vi "PH_Beckhoff_PP_PU.set i Attr and start DIM Services for PSU.vi"(0 "PU Type":T4=enum."PA 19mm", 1 "PSU Info":T1, 2 "Values":T5, 3 "error in":errorcluster) -> (6 "PSU":T3(array[cluster]) {"Status"."Status" items=["no info", "off/false/out", "on/true/in", "Failure", "Alarm", "Status 1", "Status 2", "Status 3"]}, 7 "error out":errorcluster)   [LabVIEW 2014, in "PH_Beckhoff_PP_PU.lvlib"]
uses:
  PH_Beckhoff_PP_PU.lvlib
  PH_Beckhoff/PH_Beckhoff.Values.ctl
  PH_Beckhoff/PH_Beckhoff.Sonderklemmen Inputs.ctl
  PH_Beckhoff/PH_Beckhoff.Analog Inputs.ctl
  PH_Beckhoff/PH_Beckhoff.Scaling Type.ctl
  PH_Beckhoff/PH_Beckhoff.Analog Outputs.ctl
  PH_Beckhoff/PH_Beckhoff.Digital Inputs.ctl
  PH_Beckhoff/PH_Beckhoff.Digital Outputs.ctl
  PH_Beckhoff_PP_PU.PU Rack Type.ctl
  PH_Basics/PH_StatusHandler/PH_StatusHandler.Status.ctl
  PH_Basics/PH_PP_Common/PH_PP_Common.PSU Tags.ctl
  CSlibraries-extern/DimLVEvent/LVDimInterface/LVDimInterface.lvlib
  PH_Basics/PH_StatusHandler/PH_StatusHandler.lvlib
  PH_Basics/PH_PP_Common/PH_PP_Common.lvlib
  PH_Beckhoff/PH_Beckhoff.lvlib
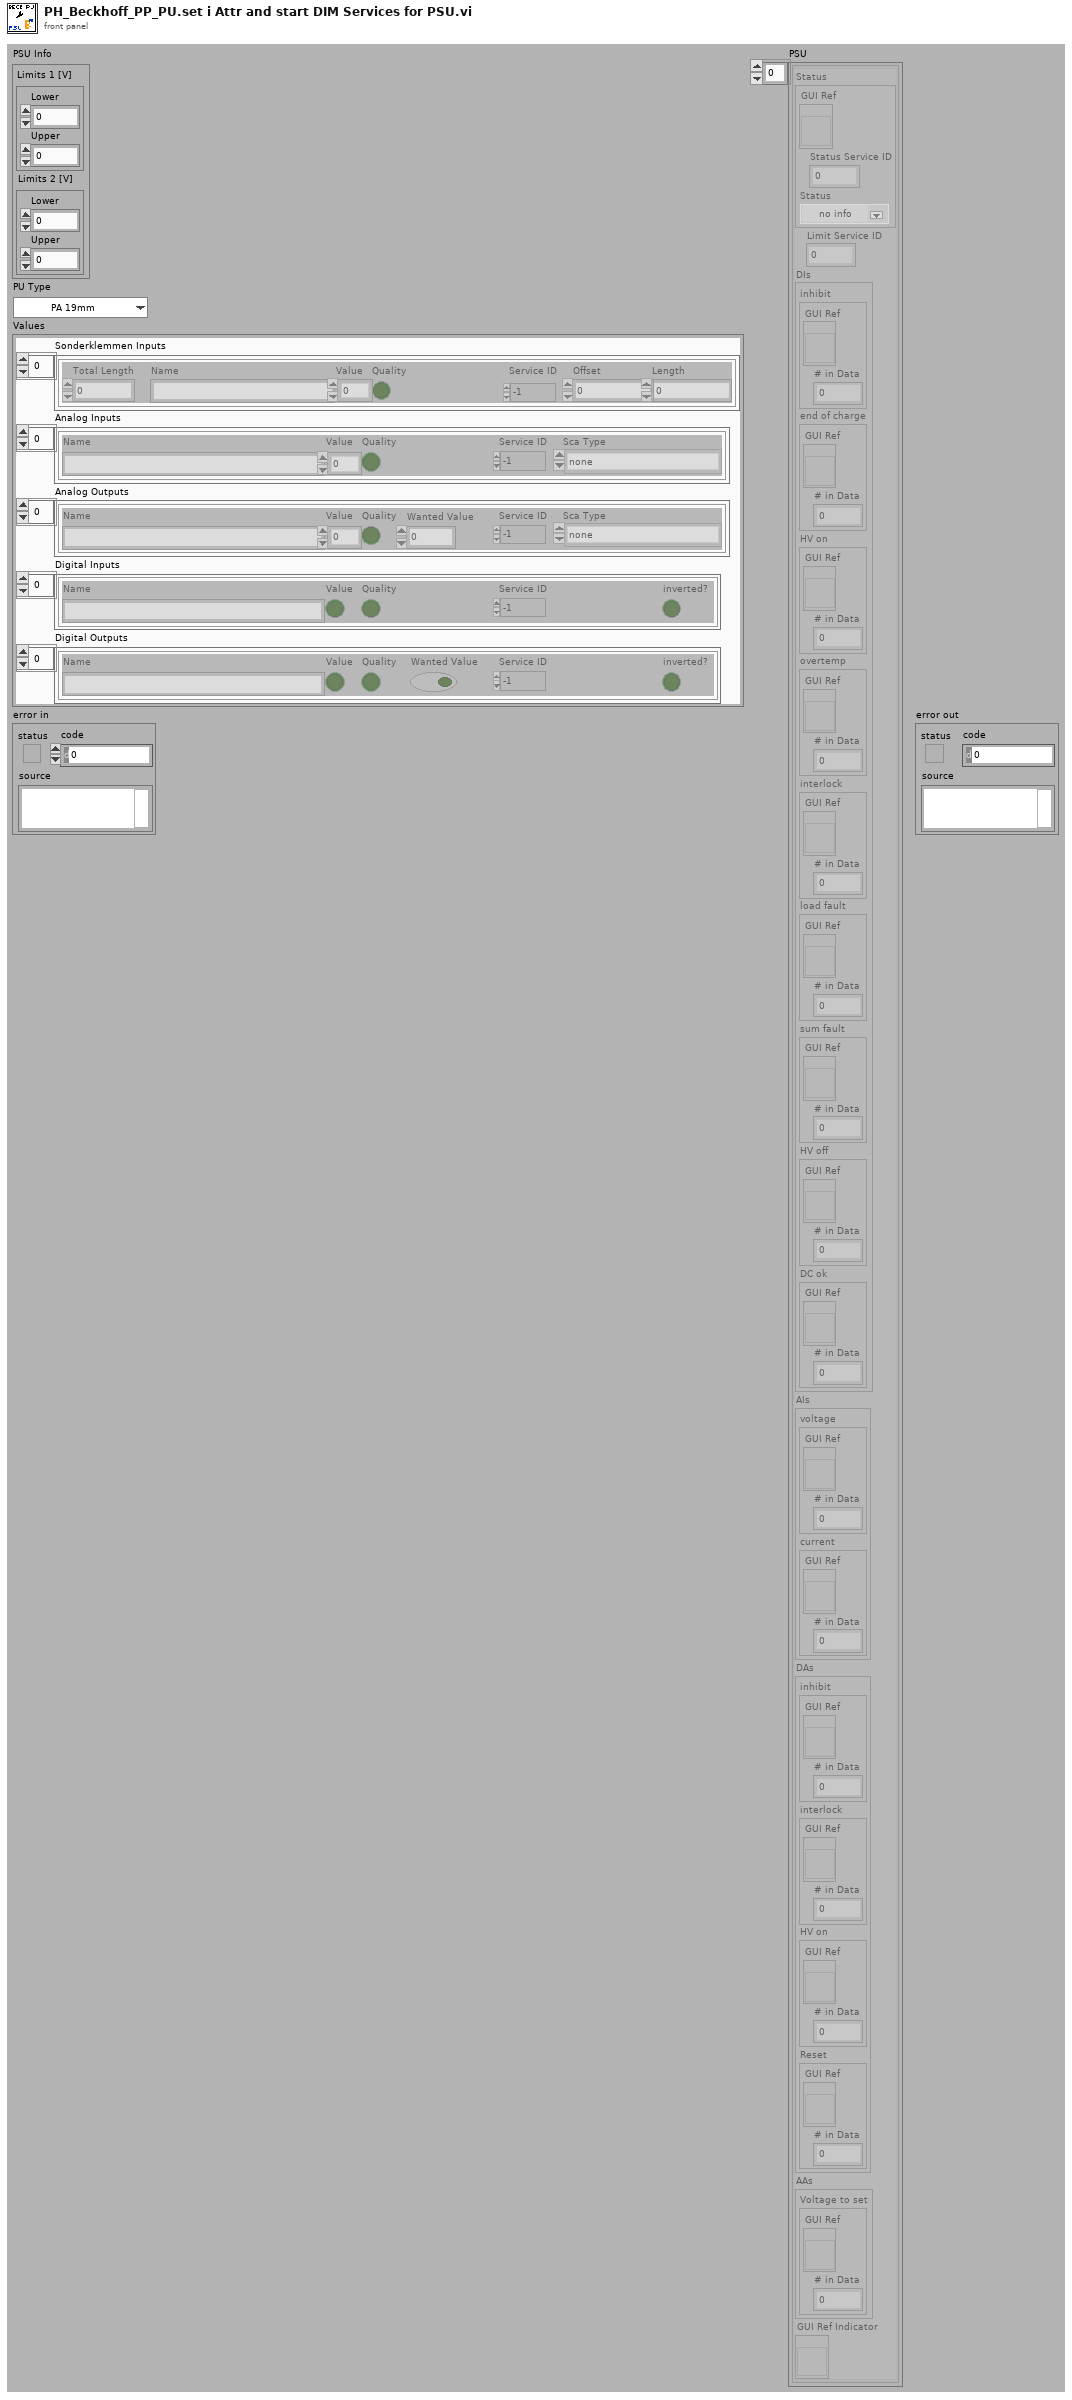
[diagram p1: front panel]
types:
  T1 = cluster{"Limits 1 [V]":cluster{"Lower":dbl, "Upper":dbl}, "Limits 2 [V]":cluster{"Lower":dbl, "Upper":dbl}}
  T2 = typedef "PH_StatusHandler.lvlib/PH_StatusHandler.Status.ctl" = i16
  T3 = cluster{"Status":cluster{"GUI Ref":refnum<vi>, "Status Service ID":i32, "Status":T2}, "Limit Service ID":i32, "DIs":cluster{"inhibit":cluster{"GUI Ref":refnum<vi>, "# in Data":i32}, "end of charge":cluster{"GUI Ref":refnum<vi>, "# in Data":i32}, "HV on":cluster{"GUI Ref":refnum<vi>, "# in Data":i32}, "overtemp":cluster{"GUI Ref":refnum<vi>, "# in Data":i32}, "interlock":cluster{"GUI Ref":refnum<vi>, "# in Data":i32}, "load fault":cluster{"GUI Ref":refnum<vi>, "# in Data":i32}, "sum fault":cluster{"GUI Ref":refnum<vi>, "# in Data":i32}, "HV off":cluster{"GUI Ref":refnum<vi>, "# in Data":i32}, "DC ok":cluster{"GUI Ref":refnum<vi>, "# in Data":i32}}, "AIs":cluster{"voltage":cluster{"GUI Ref":refnum<vi>, "# in Data":i32}, "current":cluster{"GUI Ref":refnum<vi>, "# in Data":i32}}, "DAs":cluster{"inhibit":cluster{"GUI Ref":refnum<vi>, "# in Data":i32}, "interlock":cluster{"GUI Ref":refnum<vi>, "# in Data":i32}, "HV on":cluster{"GUI Ref":refnum<vi>, "# in Data":i32}, "Reset":cluster{"GUI Ref":refnum<vi>, "# in Data":i32}}, "AAs":cluster{"Voltage to set":cluster{"GUI Ref":refnum<vi>, "# in Data":i32}}, "GUI Ref Indicator":refnum<vi>}[]
  T4 = typedef "PH_Beckhoff_PP_PU.lvlib/PH_Beckhoff_PP_PU.PU Rack Type.ctl" = enum16{"no Info", "PA 19mm", "PA 45mm", "MA PU 1 and 2", "MA PU 3 and 4", "MA PU 5 and 6", "MA FR and PILC"}
  T5 = typedef "PH_Beckhoff.lvlib/PH_Beckhoff.Values.ctl" = cluster{"Sonderklemmen Inputs":T6, "Analog Inputs":T7, "Analog Outputs":T9, "Digital Inputs":T10, "Digital Outputs":T11}
  T6 = typedef "PH_Beckhoff.lvlib/PH_Beckhoff.Sonderklemmen Inputs.ctl" = cluster{"Total Length":u32, "Name":string, "Value":u64, "Quality":bool, "Service ID":i32, "Offset":u32, "Length":u32}[]
  T7 = typedef "PH_Beckhoff.lvlib/PH_Beckhoff.Analog Inputs.ctl" = cluster{"Name":string, "Value":u32, "Quality":bool, "Service ID":i32, "Sca Type":T8}[]
  T8 = typedef "PH_Beckhoff.lvlib/PH_Beckhoff.Scaling Type.ctl" = enum16{"none", "0 ... 15 Bit -> 0 ... 5", "0 ... 15 Bit -> 0 ... 10", "0 ... 15 Bit -> 0 ... 25", "0 ... 15 Bit -> 4 ... 20", "0 ... 15 Bit -> 0 ... 1", "0 ... 15 Bit -> 0 ... 20000", "0 ... 15 Bit -> 0 ... 24000"}
  T9 = typedef "PH_Beckhoff.lvlib/PH_Beckhoff.Analog Outputs.ctl" = cluster{"Name":string, "Value":u32, "Quality":bool, "Wanted Value":u32, "Service ID":i32, "Sca Type":T8}[]
  T10 = typedef "PH_Beckhoff.lvlib/PH_Beckhoff.Digital Inputs.ctl" = cluster{"Name":string, "Value":bool, "Quality":bool, "Service ID":i32, "inverted?":bool}[]
  T11 = typedef "PH_Beckhoff.lvlib/PH_Beckhoff.Digital Outputs.ctl" = cluster{"Name":string, "Value":bool, "Quality":bool, "Wanted Value":bool, "Service ID":i32, "inverted?":bool}[]
  T12 = typedef "PH_PP_Common.lvlib/PH_PP_Common.PSU Tags.ctl" = enum16{"voltage-indicator", "peak-detect", "current", "voltage", "inihibit-indicator", "end-of-charge", "HV-on-indicator", "overtemperature", "interlock-indicator", "load-fault", "sum-fault", "HV-off-indicator", "DC-ok", "inhibit", "HV-on", "interlock", "reset", "Status", "Limits"}
  T13 = typedef "PH_PP_Common.lvlib/PH_PP_Common.PUs.ctl" = enum16{"no Info", "PA-19mm-1", "PA-19mm-2", "PA-45mm-PILC", "PA-45mm-MAIN", "MA-PU-1", "MA-PU-2", "MA-PU-3", "MA-PU-4", "MA-PU-5", "MA-PU-6", "MA-FR", "MA-PILC", "PA-45mm-DP"}
  T14 = cluster{"Status":cluster{"GUI Ref":refnum<vi>, "Status Service ID":i32, "Status":T2}, "Limit Service ID":i32, "DIs":cluster{"inhibit":cluster{"GUI Ref":refnum<vi>, "# in Data":i32}, "end of charge":cluster{"GUI Ref":refnum<vi>, "# in Data":i32}, "HV on":cluster{"GUI Ref":refnum<vi>, "# in Data":i32}, "overtemp":cluster{"GUI Ref":refnum<vi>, "# in Data":i32}, "interlock":cluster{"GUI Ref":refnum<vi>, "# in Data":i32}, "load fault":cluster{"GUI Ref":refnum<vi>, "# in Data":i32}, "sum fault":cluster{"GUI Ref":refnum<vi>, "# in Data":i32}, "HV off":cluster{"GUI Ref":refnum<vi>, "# in Data":i32}, "DC ok":cluster{"GUI Ref":refnum<vi>, "# in Data":i32}}, "AIs":cluster{"voltage":cluster{"GUI Ref":refnum<vi>, "# in Data":i32}, "current":cluster{"GUI Ref":refnum<vi>, "# in Data":i32}}, "DAs":cluster{"inhibit":cluster{"GUI Ref":refnum<vi>, "# in Data":i32}, "interlock":cluster{"GUI Ref":refnum<vi>, "# in Data":i32}, "HV on":cluster{"GUI Ref":refnum<vi>, "# in Data":i32}, "Reset":cluster{"GUI Ref":refnum<vi>, "# in Data":i32}}, "AAs":cluster{"Voltage to set":cluster{"GUI Ref":refnum<vi>, "# in Data":i32}}, "GUI Ref Indicator":refnum<vi>}
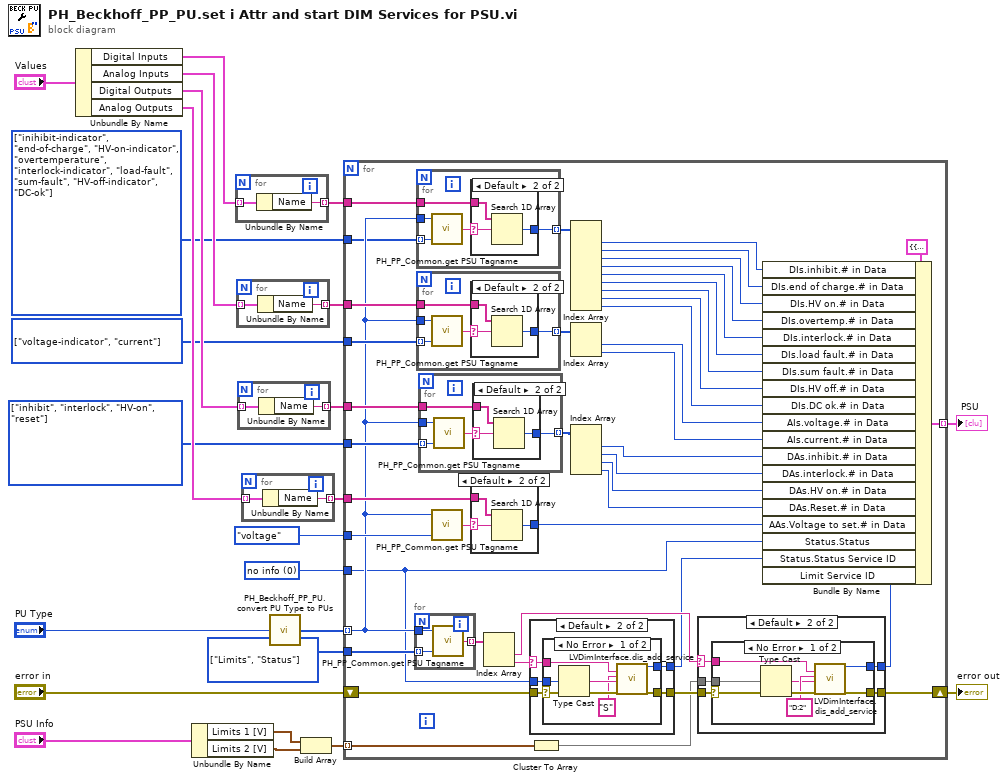
[diagram p0: block diagram]
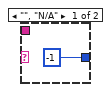
[diagram p2: hidden frame]
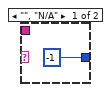
[diagram p3: hidden frame]
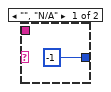
[diagram p4: hidden frame]
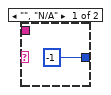
[diagram p5: hidden frame]
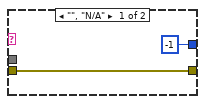
[diagram p6: hidden frame]
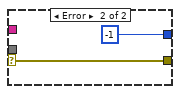
[diagram p7: hidden frame]
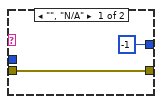
[diagram p8: hidden frame]
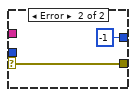
[diagram p9: hidden frame]
diagram:
  w2 = T12[] [enum."inihibit-indicator", enum."end-of-charge", enum."HV-on-indicator", enum."overtemperature", enum."interlock-indicator", enum."load-fault", enum."sum-fault", enum."HV-off-indicator", enum."DC-ok"] items=["voltage-indicator", "peak-detect", "current", "voltage", "inihibit-indicator", "end-of-charge", "HV-on-indicator", "overtemperature", "interlock-indicator", "load-fault", "sum-fault", "HV-off-indicator", "DC-ok", "inhibit", "HV-on", "interlock", "reset", "Status", "Limits"]
  w5 = T12[] [enum."voltage-indicator", enum."current"] items=["voltage-indicator", "peak-detect", "current", "voltage", "inihibit-indicator", "end-of-charge", "HV-on-indicator", "overtemperature", "interlock-indicator", "load-fault", "sum-fault", "HV-off-indicator", "DC-ok", "inhibit", "HV-on", "interlock", "reset", "Status", "Limits"]
  w8 = T12[] [enum."inhibit", enum."interlock", enum."HV-on", enum."reset"] items=["voltage-indicator", "peak-detect", "current", "voltage", "inihibit-indicator", "end-of-charge", "HV-on-indicator", "overtemperature", "interlock-indicator", "load-fault", "sum-fault", "HV-off-indicator", "DC-ok", "inhibit", "HV-on", "interlock", "reset", "Status", "Limits"]
  w14 = T12[] [enum."Limits", enum."Status"] items=["voltage-indicator", "peak-detect", "current", "voltage", "inihibit-indicator", "end-of-charge", "HV-on-indicator", "overtemperature", "interlock-indicator", "load-fault", "sum-fault", "HV-off-indicator", "DC-ok", "inhibit", "HV-on", "interlock", "reset", "Status", "Limits"]
  w19 = T2 0 items=["no info", "off/false/out", "on/true/in", "Failure", "Alarm", "Status 1", "Status 2", "Status 3"] ("Status")
  n1 = Unbundle By Name("Values") -> ("Digital Inputs"=w4:T10, "Analog Inputs"=w7:T7, "Digital Outputs"=w10:T11, "Analog Outputs"=w11:T9)
  n2 = Unbundle By Name("PSU Info") -> ("Limits 1 [V]"=w18:cluster{"Lower":dbl, "Upper":dbl}, "Limits 2 [V]"=w17:cluster{"Lower":dbl, "Upper":dbl})
  n3 = for {
    tunnel: [w25] -> w3 mode=indexing
    tunnel: w4 -> [w26] mode=indexing
    n4 = Unbundle By Name(w26) -> ("Name"=w25:string)
  }
  n5 = for {
    tunnel: [w27] -> w6 mode=indexing
    tunnel: w7 -> [w28] mode=indexing
    n6 = Unbundle By Name(w28) -> ("Name"=w27:string)
  }
  n7 = for {
    tunnel: [w29] -> w9 mode=indexing
    tunnel: w10 -> [w30] mode=indexing
    n8 = Unbundle By Name(w30) -> ("Name"=w29:string)
  }
  n9 = for {
    tunnel: [w31] -> w12 mode=indexing
    tunnel: w11 -> [w32] mode=indexing
    n10 = Unbundle By Name(w32) -> ("Name"=w31:string)
  }
  n11 = call "PH_Beckhoff_PP_PU.convert PU Type to PUs.vi"("PU Type"="PU Type") -> ("PUs"=w15:T13[])
  n12 = Build Array(w18, w17) -> (w16:cluster{"Lower":dbl, "Upper":dbl}[])
  n13 = for {
    shift-right: [w73] -> w24
    shift-left: "error in" -> [w71]
    tunnel: w19 -> [w34]
    tunnel: w16 -> [w75] mode=indexing
    tunnel: w15 -> [w36] mode=indexing
    tunnel: w14 -> [w72]
    tunnel: [w66] -> w1 mode=indexing
    tunnel: PH_PP_Common.PSU_Tags."voltage" ("PSU Tag") -> [w62]
    tunnel: w12 -> [w60]
    tunnel: w9 -> [w59]
    tunnel: w8 -> [w58]
    tunnel: w6 -> [w52]
    tunnel: w5 -> [w51]
    tunnel: w3 -> [w37]
    tunnel: w2 -> [w35]
    n14 = for {
      tunnel: w36 -> [w109]
      tunnel: w72 -> [w108] mode=indexing
      tunnel: [w107] -> w70 mode=indexing
      n15 = call "PH_PP_Common.get PSU Tagname.vi"("PSU Tag"=w108, "PU"=w109) -> ("PSU Tagname"=w107:string)  [unwired: 1 in]
    }
    n16 = for {
      tunnel: w37 -> [w79]
      tunnel: [w78] -> w47 mode=indexing
      tunnel: w35 -> [w77] mode=indexing
      tunnel: w36 -> [w76]
      n17 = call "PH_PP_Common.get PSU Tagname.vi"("PSU Tag"=w77, "PU"=w76) -> ("PSU Tagname"=w80:string)  [unwired: 1 in]
      n18 = case shown="Default" w80 {
        selector: w80 -> [_ w84]
        tunnel: [-1 ("my_serviceID") w83] -> w78
        tunnel: w79 -> [_ w82]
        frame "", "N/A" {
        }
        frame Default {
          n19 = Search 1D Array(1D array=w82, element=w84) -> (index of element=w83:i32)  [unwired: 1 in]
        }
      }
    }
    n20 = for {
      tunnel: w52 -> [w88]
      tunnel: [w87] -> w50 mode=indexing
      tunnel: w51 -> [w86] mode=indexing
      tunnel: w36 -> [w85]
      n21 = call "PH_PP_Common.get PSU Tagname.vi"("PSU Tag"=w86, "PU"=w85) -> ("PSU Tagname"=w89:string)  [unwired: 1 in]
      n22 = case shown="Default" w89 {
        selector: w89 -> [_ w93]
        tunnel: [-1 ("my_serviceID") w92] -> w87
        tunnel: w88 -> [_ w91]
        frame "", "N/A" {
        }
        frame Default {
          n23 = Search 1D Array(1D array=w91, element=w93) -> (index of element=w92:i32)  [unwired: 1 in]
        }
      }
    }
    n24 = for {
      tunnel: w59 -> [w97]
      tunnel: [w96] -> w57 mode=indexing
      tunnel: w58 -> [w95] mode=indexing
      tunnel: w36 -> [w94]
      n25 = call "PH_PP_Common.get PSU Tagname.vi"("PSU Tag"=w95, "PU"=w94) -> ("PSU Tagname"=w98:string)  [unwired: 1 in]
      n26 = case shown="Default" w98 {
        selector: w98 -> [_ w102]
        tunnel: [-1 ("my_serviceID") w101] -> w96
        tunnel: w97 -> [_ w100]
        frame "", "N/A" {
        }
        frame Default {
          n27 = Search 1D Array(1D array=w100, element=w102) -> (index of element=w101:i32)  [unwired: 1 in]
        }
      }
    }
    n28 = call "PH_PP_Common.get PSU Tagname.vi"("PSU Tag"=w62, "PU"=w36) -> ("PSU Tagname"=w63:string)  [unwired: 1 in]
    n29 = case shown="Default" w63 {
      selector: w63 -> [_ w106]
      tunnel: [-1 ("my_serviceID") w105] -> w61
      tunnel: w60 -> [_ w104]
      frame "", "N/A" {
      }
      frame Default {
        n30 = Search 1D Array(1D array=w104, element=w106) -> (index of element=w105:i32)  [unwired: 1 in]
      }
    }
    n31 = Index Array(array=w70) -> (element #1=w68:string, element #2=w69:string)  [unwired: 2 in]
    n32 = case shown="Default" w69 {
      selector: w69 -> [_ w128]
      tunnel: w71 -> [w127 w132]
      tunnel: [w127 w131] -> w74
      tunnel: [-1 ("my_serviceID") w130] -> w64
      tunnel: w34 -> [_ w129]
      frame "", "N/A" {
      }
      frame Default {
        n33 = case shown="No Error" w132 {
          selector: w132 -> [w137 w141]
          tunnel: [w139 -1 ("my_serviceID")] -> w130
          tunnel: [w138 w141] -> w131
          tunnel: w129 -> [w136 _]
          tunnel: w128 -> [w133 _]
          frame No Error {
            n34 = Type Cast(x=w136) -> (*(type *) &x=w135:string)  [unwired: 1 in]
            n35 = call "LVDimInterface.dis_add_service.vi"("serviceName"=w133, "typeDescriptor"="S", "data"=w135, "error in (no error)"=w137) -> ("my_serviceID"=w139:i32, "error out"=w138:errorcluster)  [unwired: 14 in]
          }
          frame Error {
          }
        }
      }
    }
    n36 = Cluster To Array(cluster=w75) -> (array=w67:dbl[])
    n37 = Index Array(array=w47) -> (element #1=w46:i32, element #2=w45:i32, element #3=w44:i32, element #4=w43:i32, element #5=w42:i32, element #6=w41:i32, element #7=w40:i32, element #8=w39:i32, element #9=w38:i32)  [unwired: 9 in]
    n38 = Index Array(array=w50) -> (element #1=w48:i32, element #2=w49:i32)  [unwired: 2 in]
    n39 = Index Array(array=w57) -> (element #1=w56:i32, element #2=w55:i32, element #3=w54:i32, element #4=w53:i32)  [unwired: 4 in]
    n40 = case shown="Default" w68 {
      selector: w68 -> [_ w112]
      tunnel: [-1 ("my_serviceID") w116] -> w65
      tunnel: w67 -> [_ w115]
      tunnel: w74 -> [w110 w114]
      tunnel: [w110 w113] -> w73
      frame "", "N/A" {
      }
      frame Default {
        n41 = case shown="No Error" w114 {
          selector: w114 -> [w122 w125]
          tunnel: [w118 -1 ("my_serviceID")] -> w116
          tunnel: [w123 w125] -> w113
          tunnel: w115 -> [w117 _]
          tunnel: w112 -> [w120 _]
          frame No Error {
            n42 = Type Cast(x=w117) -> (*(type *) &x=w119:string)  [unwired: 1 in]
            n43 = call "LVDimInterface.dis_add_service.vi"("serviceName"=w120, "typeDescriptor"="D:2", "data"=w119, "error in (no error)"=w122) -> ("my_serviceID"=w118:i32, "error out"=w123:errorcluster)  [unwired: 14 in]
          }
          frame Error {
          }
        }
      }
    }
    n44 = Bundle By Name(cluster=T14 {"Status"={"GUI Ref"=refnum, "Status Service ID"=0, "Status"=0}, "Limit Service ID"=0, "DIs"={"inhibit"={"GUI Ref"=refnum, "# in Data"=0}, "end of charge"={"GUI Ref"=refnum, "# in Data"=0}, "HV on"={"GUI Ref"=refnum, "# in Data"=0}, "overtemp"={"GUI Ref"=refnum, "# in Data"=0}, "interlock"={"GUI Ref"=refnum, "# in Data"=0}, "load fault"={"GUI Ref"=refnum, "# in Data"=0}, "sum fault"={"GUI Ref"=refnum, "# in Data"=0}, "HV off"={"GUI Ref"=refnum, "# in Data"=0}, "DC ok"={"GUI Ref"=refnum, "# in Data"=0}}, "AIs"={"voltage"={"GUI Ref"=refnum, "# in Data"=0}, "current"={"GUI Ref"=refnum, "# in Data"=0}}, "DAs"={"inhibit"={"GUI Ref"=refnum, "# in Data"=0}, "interlock"={"GUI Ref"=refnum, "# in Data"=0}, "HV on"={"GUI Ref"=refnum, "# in Data"=0}, "Reset"={"GUI Ref"=refnum, "# in Data"=0}}, "AAs"={"Voltage to set"={"GUI Ref"=refnum, "# in Data"=0}}, "GUI Ref Indicator"=refnum} ("PSU Data"), "DIs.inhibit.# in Data"=w46, "DIs.end of charge.# in Data"=w45, "DIs.HV on.# in Data"=w44, "DIs.overtemp.# in Data"=w43, "DIs.interlock.# in Data"=w42, "DIs.load fault.# in Data"=w41, "DIs.sum fault.# in Data"=w40, "DIs.HV off.# in Data"=w39, "DIs.DC ok.# in Data"=w38, "AIs.voltage.# in Data"=w48, "AIs.current.# in Data"=w49, "DAs.inhibit.# in Data"=w56, "DAs.interlock.# in Data"=w55, "DAs.HV on.# in Data"=w54, "DAs.Reset.# in Data"=w53, "AAs.Voltage to set.# in Data"=w61, "Status.Status"=w34, "Status.Status Service ID"=w64, "Limit Service ID"=w65) -> (w66:T14)
  }
  "error out" <- w24
  "PSU" <- w1
